vi "UpdateNotes.vi"(8 "error in (no error)":errorcluster, 9 "Scan Key":T1, 10 "reference":refnum<vi>, 11 "Database in":refnum<class "Database.lvclass">) -> (0 "error out":errorcluster, 3 "Database out":refnum<class "Database.lvclass">)   [LabVIEW 2014, in "Database.lvclass"]
uses:
  Database.lvclass
  Database.lvclass/Database.ctl
  <vilib>/addons/database/NI_Database_API.lvlib
panel:
  out "Value":variant
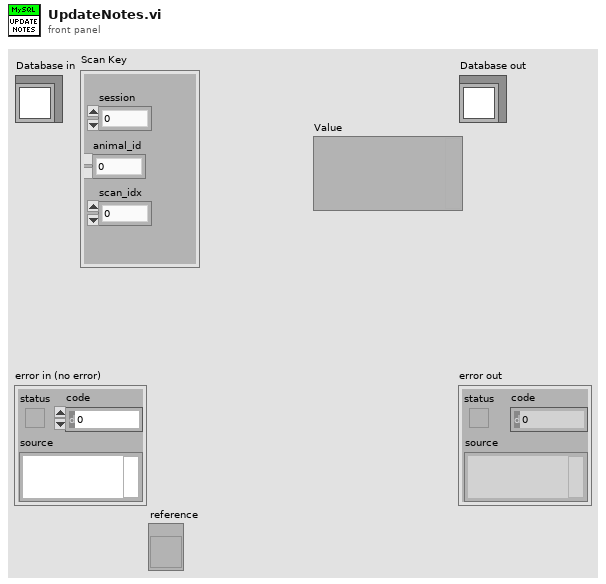
[diagram p1: front panel]
types:
  T1 = cluster{"session":dbl, "animal_id":dbl, "scan_idx":dbl}
  T2 = typedef "NI_Database_API.lvlib/Conn ObjectReference.ctl" = refnum<k1>
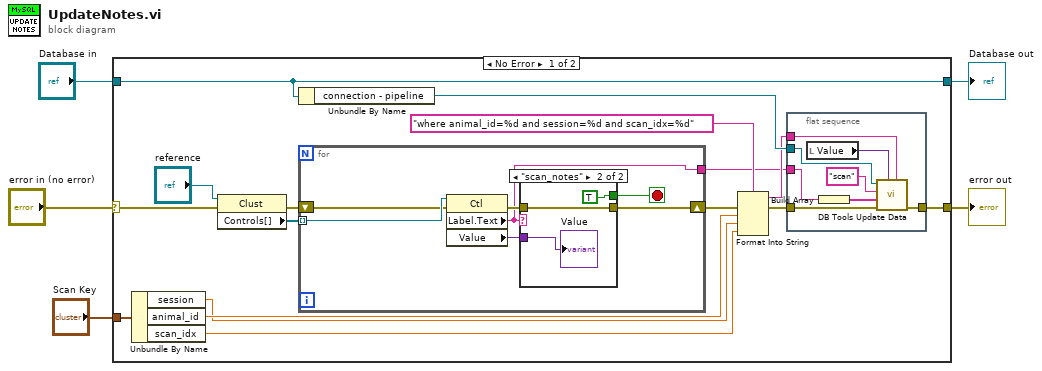
[diagram p0: block diagram]
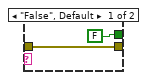
[diagram p2: hidden frame]
diagram:
  n1 = case shown="No Error" "error in (no error)" {
    selector: "error in (no error)" -> [w19 w43]
    tunnel: [w15 w43] -> w4
    tunnel: [w21 w42] -> w2
    tunnel: "Database in" -> [w21 w42]
    tunnel: "Scan Key" -> [w10 _]
    frame No Error {
      n2 = Unbundle By Name(w10) -> ("session"=w8:dbl, "animal_id"=w9:dbl, "scan_idx"=w7:dbl)
      n3 = property class="Clust"(reference="reference", error in=w19) -> (error out=w17:errorcluster, "Controls[]"=w18:refnum<vi>[])  [unwired: 1 out]
      n4 = Unbundle By Name(w21) -> ("connection - pipeline"=w16:T2)
      n5 = for {
        tunnel: w18 -> [w36] mode=indexing
        shift-right: [w31] -> w12
        shift-left: w17 -> [w33]
        tunnel: [w30] -> w6
        stop <- w35 stop-if-true
        n6 = property class="Ctl"(reference=w36, error in=w33) -> (error out=w32:errorcluster, "Label.Text"=w30:string, "Value"=w34:variant)  [unwired: 1 out]
        n7 = case shown="\"scan_notes\"" w30 {
          tunnel: [FALSE TRUE] -> w35
          tunnel: w34 -> [_ w40]
          tunnel: w32 -> [w37 w39]
          tunnel: [w37 w39] -> w31
          frame "False", Default {
          }
          frame "scan_notes" {
            "Value" <- w40
          }
        }
      }
      n8 = Format Into String(format string="where animal_id=%d and session=%d and scan_idx=%d", error in=w12, w9, w8, w7) -> (resulting string=w13:string, error out=w11:errorcluster)  [unwired: 1 in]
      n9 = flat-sequence {
        tunnel: w11 -> [w27]
        tunnel: w16 -> [w29]
        tunnel: [w26] -> w15
        tunnel: w13 -> [w24]
        tunnel: w6 -> [w23]
        frame #0 {
          n10 = local read "Value"() -> (w25:variant)
          n11 = Build Array(w23) -> (w22:string[])
          n12 = call <vilib>:"DB Tools Update Data.vi"("condition"=w24, "data"=w25, "error in (no error)"=w27, "columns"=w22, "table"="scan", "connection reference"=w29) -> ("error out"=w26:errorcluster)  [unwired: 4 in, 1 out]
        }
      }
    }
    frame Error {
    }
  }
  "error out" <- w4
  "Database out" <- w2
